vi "P3-2.vi"() -> ()   [LabVIEW 2011]
panel:
  out "NOT Z":bool
  out "X OR Y":bool
  out "X AND Y":bool
  in  "Z":bool
  in  "Y":bool
  in  "X":bool
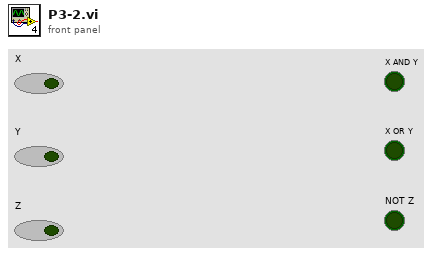
[diagram p1: front panel]
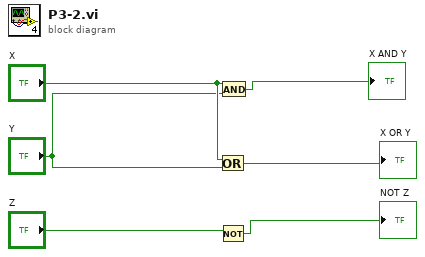
[diagram p0: block diagram]
diagram:
  n1 = Or(x="X", y="Y") -> (x .or. y?=→"X OR Y":bool)
  n2 = Not(x="Z") -> (.not. x?=→"NOT Z":bool)
  n3 = And(x="X", y="Y") -> (x .and. y?=→"X AND Y":bool)
